vi "Read Spreadsheet File with Path Validation.vi"(0 "Path In":path, 1 "format (%s)":string="%s", 2 "Expected File Extention":string[](array[string])=["csv", "txt"], 5 "number of rows (all:-1)":i32=-1, 7 "start of read offset (chars.:0)":i32, 9 "max characters/row  (no limit:0)":i32, 11 "error in (no error)":errorcluster, 12 "transpose (no:F)":bool, 13 "delimiter (\\t)":string="\t") -> (4 "Path Out":path, 6 "all rows":string[][](array[string]), 8 "first row":string[](array[string]), 10 "mark after read (chars.)":i32=-1, 14 "EOF?":bool, 15 "error out":errorcluster)   [LabVIEW 2014]
uses:
  <vilib>/Utility/file.llb/Read From Spreadsheet File (string).vi
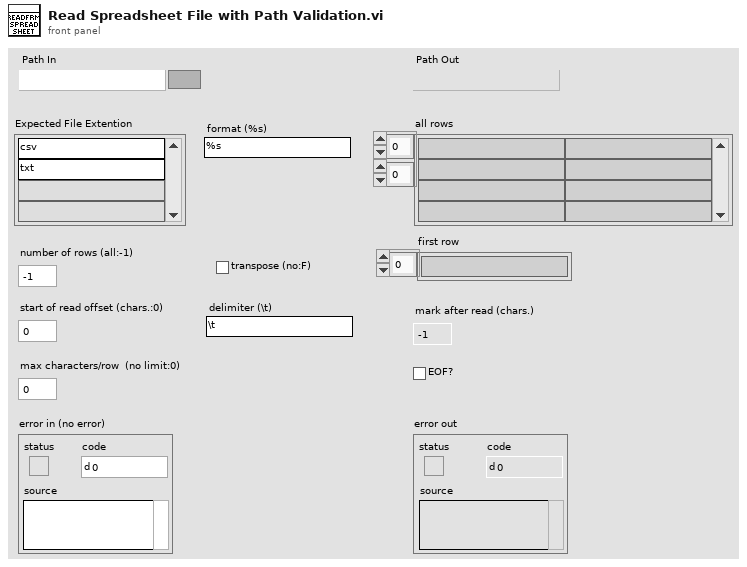
[diagram p1: front panel]
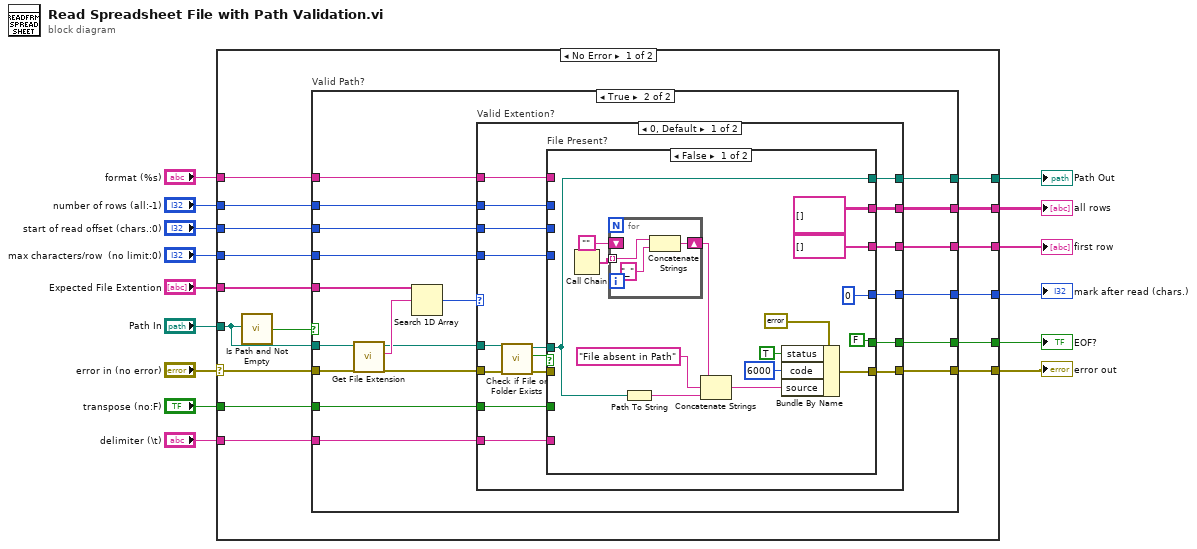
[diagram p0: block diagram]
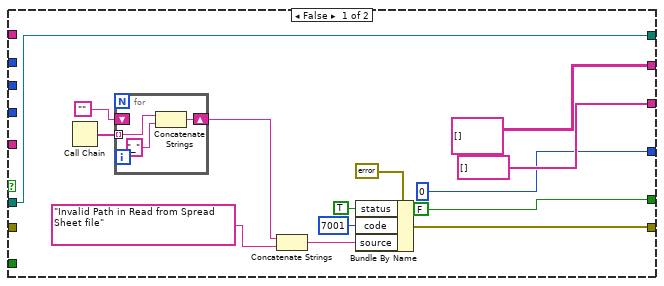
[diagram p2: hidden frame]
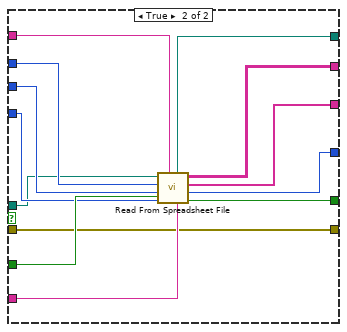
[diagram p3: hidden frame]
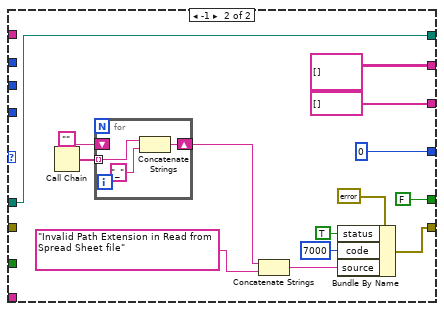
[diagram p4: hidden frame]
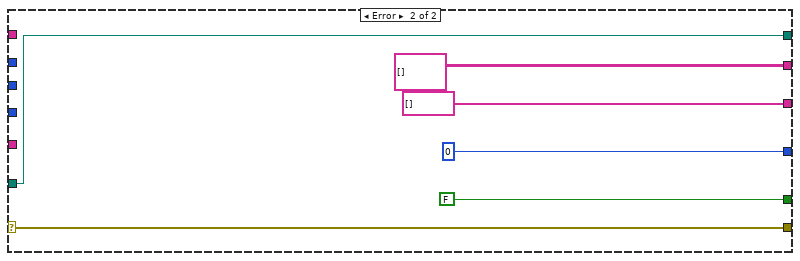
[diagram p5: hidden frame]
diagram:
  n1 = case shown="No Error" "error in (no error)" {
    selector: "error in (no error)" -> [w30 w138]
    tunnel: "Path In" -> [w29 w135]
    tunnel: "Expected File Extention" -> [w28 _]
    tunnel: [w27 w138] -> w12
    tunnel: "format (%s)" -> [w26 _]
    tunnel: [w25 w135] -> w10
    tunnel: [w24 string[][] [] ("all rows")] -> w4
    tunnel: [w23 string[] [] ("first row")] -> w2
    tunnel: [w22 0 ("mark after read (chars.)")] -> w1
    tunnel: [w21 FALSE ("EOF?")] -> w3
    tunnel: "delimiter (\\t)" -> [w20 _]
    tunnel: "transpose (no:F)" -> [w19 _]
    tunnel: "number of rows (all:-1)" -> [w18 _]
    tunnel: "start of read offset (chars.:0)" -> [w17 _]
    tunnel: "max characters/row  (no limit:0)" -> [w16 _]
    frame No Error {
      n2 = call <vilib>:"Is Path and Not Empty.vi"("path"=w29) -> ("Is Path and Not Empty?"=w31:bool)  [unwired: 4 in]
      n3 = case "Valid Path?" shown="True" w31 {
        tunnel: w30 -> [_ w67]
        tunnel: w29 -> [w45 w66]
        tunnel: w28 -> [_ w65]
        tunnel: [w32 w49] -> w27
        tunnel: w26 -> [_ w61]
        tunnel: [w45 w60] -> w25
        tunnel: [string[][] [] ("all rows") w59] -> w24
        tunnel: [string[] [] ("first row") w58] -> w23
        tunnel: [0 ("mark after read (chars.)") w57] -> w22
        tunnel: [FALSE ("EOF?") w56] -> w21
        tunnel: w20 -> [_ w55]
        tunnel: w19 -> [_ w54]
        tunnel: w18 -> [_ w53]
        tunnel: w17 -> [_ w52]
        tunnel: w16 -> [_ w51]
        frame False {
          n4 = Call Chain() -> (call chain=w40:string[])
          n5 = for {
            tunnel: w40 -> [w48] mode=indexing
            shift-right: [w46] -> w35
            shift-left: "" -> [_]
            n6 = Concatenate Strings(w48, "_" ("string")) -> (w46:string)
          }
          n7 = Concatenate Strings(w35, "Invalid Path in Read from Spread Sheet file" ("string")) -> (w33:string)
          n8 = Bundle By Name(cluster=errorcluster {"status"=FALSE, "code"=0, "source"=""} ("error in (no error)"), "status"=TRUE, "code"=7001, "source"=w33) -> (w32:errorcluster)
        }
        frame True {
          n9 = call <vilib>:"Get File Extension.vi"("error in (no error)"=w67, "file"=w66) -> ("error out"=w50:errorcluster, "lowercase file extension"=w64:string, "dup file"=w62:path)  [unwired: 6 in, 1 out]
          n10 = Search 1D Array(1D array=w65, element=w64) -> (index of element=w63:i32)  [unwired: 1 in]
          n11 = case "Valid Extention?" shown="0, Default" w63 {
            tunnel: w62 -> [w72 w129]
            tunnel: w61 -> [w84 _]
            tunnel: [w83 w129] -> w60
            tunnel: [w82 string[][] [] ("all rows")] -> w59
            tunnel: [w81 string[] [] ("first row")] -> w58
            tunnel: [w80 0 ("mark after read (chars.)")] -> w57
            tunnel: [w79 FALSE ("EOF?")] -> w56
            tunnel: w55 -> [w78 _]
            tunnel: w54 -> [w77 _]
            tunnel: w53 -> [w76 _]
            tunnel: w52 -> [w75 _]
            tunnel: w51 -> [w74 _]
            tunnel: w50 -> [w73 _]
            tunnel: [w68 w118] -> w49
            frame 0, Default {
              n12 = call <vilib>:"Check if File or Folder Exists.vi"("error in (no error)"=w73, "path"=w72) -> ("error out"=w70:errorcluster, "file or folder exists?"=w69:bool, "dup path"=w71:path)  [unwired: 7 in]
              n13 = case "File Present?" shown="False" w69 {
                tunnel: w84 -> [_ w115]
                tunnel: [w85 w114] -> w83
                tunnel: [string[][] [] ("all rows") w113] -> w82
                tunnel: [string[] [] ("first row") w112] -> w81
                tunnel: [0 ("mark after read (chars.)") w111] -> w80
                tunnel: [FALSE ("EOF?") w110] -> w79
                tunnel: w78 -> [_ w109]
                tunnel: w77 -> [_ w108]
                tunnel: w76 -> [_ w107]
                tunnel: w75 -> [_ w106]
                tunnel: w74 -> [_ w105]
                tunnel: w71 -> [w85 w104]
                tunnel: w70 -> [_ w103]
                tunnel: [w94 w103] -> w68
                frame False {
                  n14 = Call Chain() -> (call chain=w98:string[])
                  n15 = for {
                    tunnel: w98 -> [w102] mode=indexing
                    shift-right: [w100] -> w92
                    shift-left: "" -> [_]
                    n16 = Concatenate Strings(w102, "_" ("string")) -> (w100:string)
                  }
                  n17 = Path To String(path=w85) -> (string=w93:string)
                  n18 = Concatenate Strings(w92, "File absent in Path" ("string"), w93) -> (w90:string)
                  n19 = Bundle By Name(cluster=errorcluster {"status"=FALSE, "code"=0, "source"=""} ("error in (no error)"), "status"=TRUE, "code"=6000, "source"=w90) -> (w94:errorcluster)
                }
                frame True {
                  n20 = call-poly <vilib>:"Read From Spreadsheet File.vi"("delimiter (\\t)"=w109, "transpose (no:F)"=w108, "format (%s)"=w115, "max characters/row  (no limit:0)"=w105, "start of read offset (chars.:0)"=w106, "number of rows (all:-1)"=w107, "file path (dialog if empty)"=w104) -> ("EOF?"=w110:bool, "mark after read (chars.)"=w111:i32, "first row"=w112:string[], "all rows"=w113:string[][], "new file path (Not A Path if cancelled)"=w114:path)
                }
              }
            }
            frame -1 {
              n21 = Call Chain() -> (call chain=w126:string[])
              n22 = for {
                tunnel: w126 -> [w132] mode=indexing
                shift-right: [w130] -> w121
                shift-left: "" -> [_]
                n23 = Concatenate Strings(w132, "_" ("string")) -> (w130:string)
              }
              n24 = Concatenate Strings(w121, "Invalid Path Extension in Read from Spread Sheet file" ("string")) -> (w119:string)
              n25 = Bundle By Name(cluster=errorcluster {"status"=FALSE, "code"=0, "source"=""} ("error in (no error)"), "status"=TRUE, "code"=7000, "source"=w119) -> (w118:errorcluster)
            }
          }
        }
      }
    }
    frame Error {
    }
  }
  "error out" <- w12
  "Path Out" <- w10
  "all rows" <- w4
  "first row" <- w2
  "mark after read (chars.)" <- w1
  "EOF?" <- w3
